vi "is_inside.vi"(8 "error in (no error)":errorcluster, 10 "SpaceVector.lvclass":refnum<class "SpaceVector.lvclass">, 11 "ROI in":refnum<class "RoiGeneric.lvclass">) -> (0 "error out":errorcluster, 2 "is inside?":bool, 3 "ROI out":refnum<class "RoiGeneric.lvclass">)   [LabVIEW 2010, in "RoiGeneric.lvclass"]
uses:
  RoiGeneric.lvclass
  common/classes/SpaceVector/SpaceVector/SpaceVector.lvclass
  common/classes/Box/Box/Box.lvclass
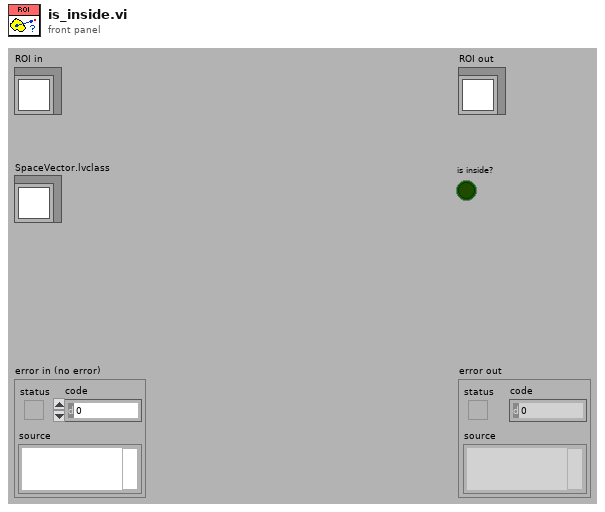
[diagram p1: front panel]
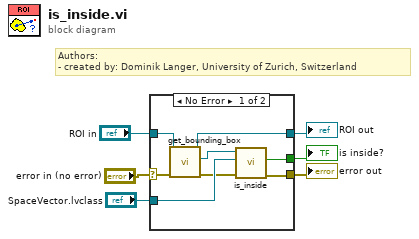
[diagram p0: block diagram]
diagram:
  # "Authors: \n- created by: Dominik Langer, University of Zurich, Switzerland"
  n1 = case shown="No Error" "error in (no error)" {
    selector: "error in (no error)" -> [w12 w16]
    tunnel: [w7 w16] -> w5
    tunnel: [w13 w15] -> w3
    tunnel: "ROI in" -> [w14 w15]
    tunnel: [w8 _] -> w2
    tunnel: "SpaceVector.lvclass" -> [w11 _]
    frame No Error {
      n2 = call-dynamic "get_bounding_box.vi"("error in (no error)"=w12, "RoiGeneric in"=w14) -> ("error out"=w10:errorcluster, "Box.lvclass"=w9:refnum<class "Box.lvclass">, "RoiGeneric out"=w13:refnum<class "RoiGeneric.lvclass">)  [unwired: 7 in]
      n3 = call "is_inside.vi"("error in (no error)"=w10, "SpaceVector.lvclass"=w11, "Box in"=w9) -> ("error out"=w7:errorcluster, "is inside?"=w8:bool)  [unwired: 6 in, 1 out]
    }
    frame Error {
    }
  }
  "error out" <- w5
  "ROI out" <- w3
  "is inside?" <- w2
